vi "Ophir SendPower.vi"(0 "Visa Session":refnum<visa-resource-name>, 1 "error in (no error)":errorcluster) -> (2 "dup Visa Session":refnum<visa-resource-name>, 3 "Value Number":dbl format="%.3e", 4 "Value String":string, 5 "error out":errorcluster)   [LabVIEW 2017]
doc: "SendPower.vi returns power measurement from instrument.\nVersion 1.00 \nLast Updated 16 March 2005\n\nThe VI doesn't include the Power Configuration Initialization\nof the Device.\n\nInputs:\nVisa Session\nErrorIn\n\nOutputs:\ndup Visa Session\nValue Number is the measurement value\nValue String is the measurement string\n\nNote:\nIn case of Overrange Measure The string contains *OVER\nErrorOut\nReturns Error n# -1339 when Measurement Failed"
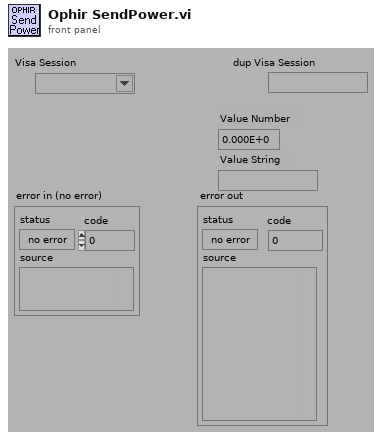
[diagram p1: front panel]
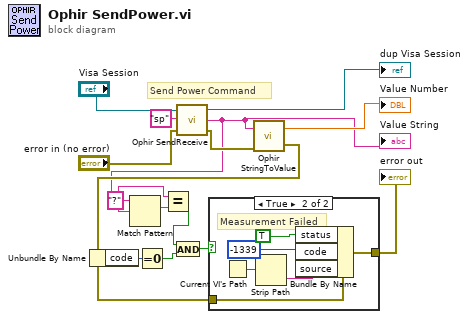
[diagram p0: block diagram]
diagram:
  w5 = "?"
  # "Send Power Command"
  n1 = call "Ophir SendReceive.vi"("error in (no error)"="error in (no error)", "Command"="sp", "Visa Session"="Visa Session") -> ("error out"=w11:errorcluster, "Frame Output"=w4:string, "dup Visa Session"=→"dup Visa Session":refnum<visa-resource-name>)
  "Value String" <- w4
  n2 = Match Pattern(string=w4, regular expression=w5) -> (match substring=w3:string)  [unwired: 4 out]
  n3 = Equal?(x=w5, y=w3) -> (x = y?=w2:bool)
  n4 = call "Ophir StringToValue.vi"("error in (no error)"=w11, "Frame"=w4) -> ("error out"=w9:errorcluster, "Value"=→"Value Number":dbl)
  n5 = Unbundle By Name(w9) -> ("code"=w7:i32)
  n6 = Equal To 0?(x=w7) -> (x = 0?=w6:bool)
  n7 = And(x=w2, y=w6) -> (x .and. y?=w1:bool)
  n8 = case shown="True" w1 {
    tunnel: w9 -> [w16 w19]
    tunnel: [w16 w18] -> w8
    frame False {
      # "No Error or \nError already exists"
    }
    frame True {
      # "Measurement Failed"
      n9 = Current VI's Path() -> (path=w17:path)
      n10 = Strip Path(path=w17) -> (name=w20:string)  [unwired: 1 out]
      n11 = Bundle By Name(cluster=w19, "status"=TRUE, "code"=-1339, "source"=w20) -> (w18:errorcluster)
    }
  }
  "error out" <- w8
